vi "Rotation Globals.vi"() -> ()   [LabVIEW 2016]
uses:
  Rotation Notifier.ctl
  Rotation Control Type.ctl
panel:
  out "Up":bool
  in  "Position":dbl
  in  "Positional Motor":string="Positional Motor"
  in  "Rotation DVR":refnum<data-value>
  in  "Rotation Notifier":refnum<notifier>
  # "These refnums are for the writing and creation\nof the rotation subsystem's data."
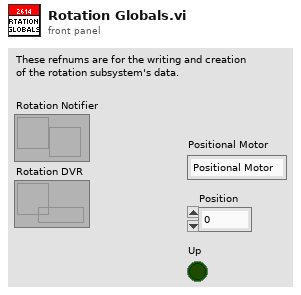
[diagram p1: front panel]
diagram:
